vi "daqio_Get_Device_Waveforms.vi"(6 "End Time":timestamp, 7 "Start Time":timestamp, 8 "error in":errorcluster, 10 "Channel Name":string, 11 "daq.io type in":T1={"daq.io ref"=refnum, "daq.io API Base"="http://dashboard.daq.io/api/v1", "Device Type Key"="", "Device Key"="", "Account ID"="", "online"=TRUE, "SSL"=TRUE}) -> (0 "error out":errorcluster, 1 "Waveform Labels":string[](array[string]), 2 "Waveforms":waveform(dbl)[](array[waveform]), 3 "daq.io type out":T1={"daq.io ref"=refnum, "daq.io API Base"="http://dashboard.daq.io/api/v1", "Device Type Key"="", "Device Key"="", "Account ID"="", "online"=TRUE, "SSL"=TRUE})   [LabVIEW 2013, in "daqio minimal.lvlib"]
doc: "This VI returns all Events for a specific Device."
uses:
  daqio minimal.lvlib
  _typedefs/daqio-Type.ctl
  <vilib>/httpClient/ClientHandle.ctl
  <vilib>/httpClient/LabVIEWHTTPClient.lvlib
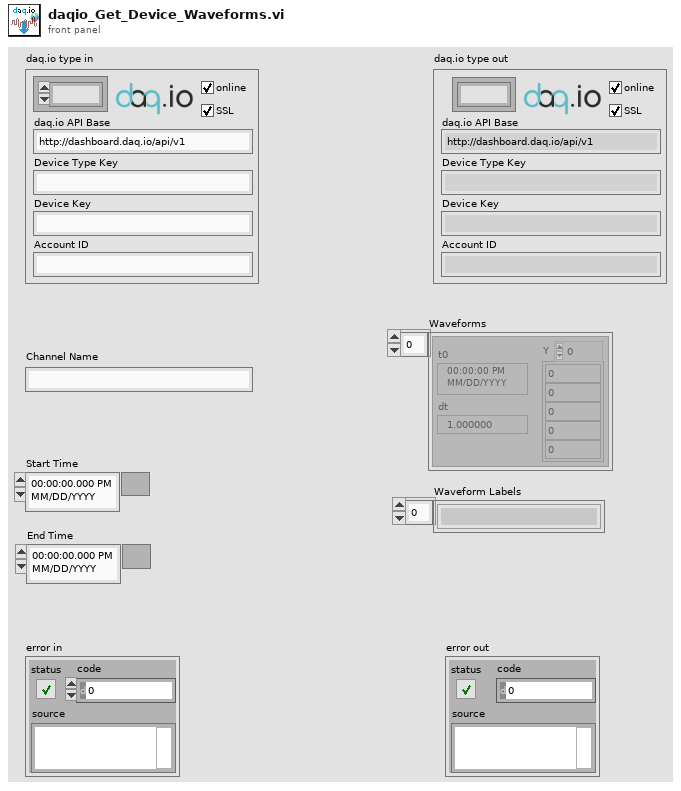
[diagram p1: front panel]
types:
  T1 = typedef "daqio minimal.lvlib/daqio-Type.ctl" = cluster{"daq.io ref":T2, "daq.io API Base":string, "Device Type Key":string, "Device Key":string, "Account ID":string, "online":bool, "SSL":bool}
  T2 = typedef "LabVIEWHTTPClient.lvlib/ClientHandle.ctl" = refnum<k1>
  T3 = typedef "daqio minimal.lvlib/daqio-read-waveform-JSON-header-time.ctl" = cluster{"id":string, "label":string, "channel_type_id":string, "device_id":string, "start_time":timestamp}
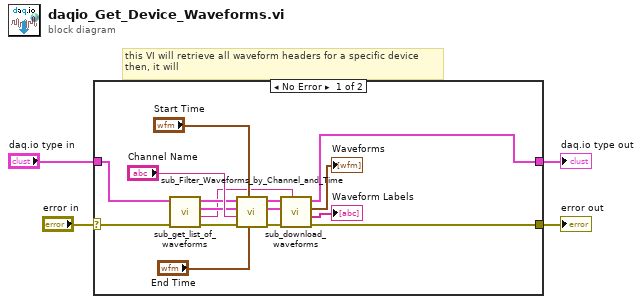
[diagram p0: block diagram]
diagram:
  # "this VI will retrieve all waveform headers for a specific device\nthen, it will"
  n1 = case shown="No Error" "error in" {
    selector: "error in" -> [w11 w21]
    tunnel: "daq.io type in" -> [w9 w22]
    tunnel: [w5 w22] -> w3
    tunnel: [w7 w21] -> w2
    frame No Error {
      n2 = call "sub_get_list_of_waveforms.vi"("error in"=w11, "daq.io type in"=w9) -> ("error out"=w15:errorcluster, "Waveform base URI"=w6:string, "Existing Waveforms"=w12:T3[], "daq.io type out"=w10:T1)  [unwired: 6 in]
      n3 = call "sub_Filter_Waveforms_by_Channel_and_Time.vi"("End Time"="End Time", "Start Time"="Start Time", "error in"=w15, "Channel Key"="Channel Name", "Waveforms in"=w12, "daq.io type in"=w10) -> ("error out"=w14:errorcluster, "Filtered Waveforms out"=w13:T3[], "daq.io type out"=w8:T1)  [unwired: 3 in]
      n4 = call "sub_download_waveforms.vi"("Waveform base URI"=w6, "error in"=w14, "Filtered Waveforms in"=w13, "daq.io type in"=w8) -> ("error out"=w7:errorcluster, "Waveform Labels out"=→"Waveform Labels":string[], "Waveform Data out"=→"Waveforms":waveform(dbl)[], "daq.io type out"=w5:T1)  [unwired: 3 in, 1 out]
    }
    frame Error {
    }
  }
  "error out" <- w2
  "daq.io type out" <- w3
